vi "GetPublicEvents.vi"(8 "error in (no error)":errorcluster, 11 "SMO":refnum<class "SMO.lvclass">) -> (0 "error out":errorcluster, 2 "Public Events":T1, 3 "SMO out":refnum<class "SMO.lvclass">)   [LabVIEW 2013, in "SMO.lvclass"]
uses:
  SMO.lvclass
  Typedefs/Public Events.ctl
  SMO.lvclass/SMO.ctl
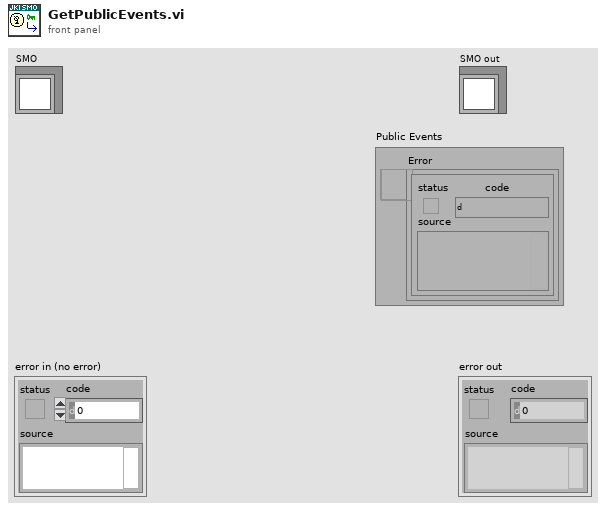
[diagram p1: front panel]
types:
  T1 = typedef "SMO.lvclass/Public Events.ctl" = cluster{"Error":refnum<user-event>}
  T2 = typedef "SMO.lvclass/PrivateData--Ref.ctl" = refnum<data-value>
  T3 = typedef "SMO.lvclass/PrivateData--Cluster.ctl" = cluster{"SMO Name":string, "Parent Call":T4, "Registered Processes":T5[], "Process Sync RendezVous":T6, "Process Error Notifier":refnum<notifier>, "Protected Events":T7, "Public Events":T1}
  T4 = typedef "SMO.lvclass/Parent Call--Enum.ctl" = enum16{"Allows parent to run", "Does not request parent to run"}
  T5 = typedef "SMO.lvclass/RegisteredProcessData--Cluster.ctl" = cluster{"Name":string, "Static VI Ref":refnum<vi>, "Running":bool}
  T6 = typedef "Rendezvous RefNum" = refnum<k1>
  T7 = typedef "SMO.lvclass/Protected Events.ctl" = cluster{"StopProcesses":refnum<user-event>, "AbortProcesses":refnum<user-event>}
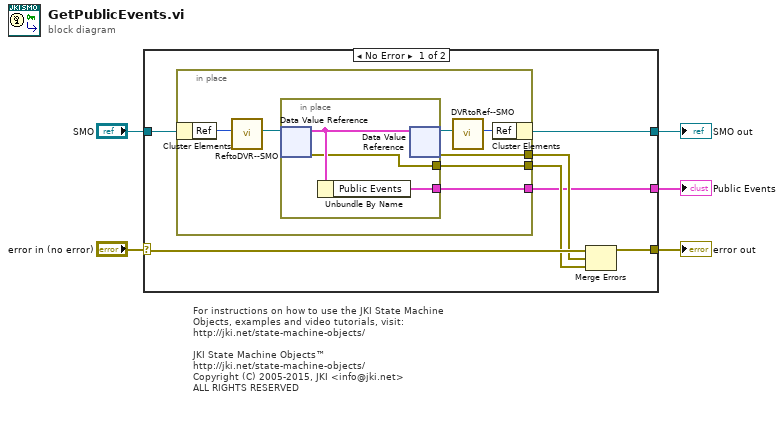
[diagram p0: block diagram]
diagram:
  # "For instructions on how to use the JKI State Machine Objects, examples and video tutorials, visit:\nhttp://jki.net/state-machine-objects/\n\nJKI State Machine Objects™\nhttp://jki.net/state-machine-objects/\nCopyright (C) 2005-2015, JKI <info@jki.net>\nALL RIGHTS RESERVED"
  n1 = case shown="No Error" "error in (no error)" {
    selector: "error in (no error)" -> [w10 w24]
    tunnel: [w9 w24] -> w4
    tunnel: [w11 w23] -> w2
    tunnel: "SMO" -> [w12 w23]
    tunnel: [w6 _] -> w1
    frame No Error {
      n2 = in-place {
        in-place-border: [w19] -> w6
        in-place-border: [w18] -> w8
        in-place-border: [w17] -> w7
        n3 = in-place-cluster #1(w12) -> ("Ref"=w16:u32)
        n4 = call "ReftoDVR--SMO.vi"("Ref"=w16) -> ("Ref"=w15:T2)  [unwired: 10 in]
        n5 = in-place {
          in-place-border: [w22] -> w19
          in-place-border: [w20] -> w17
          n6 = in-place-dvr #2(w15) -> (w21:T3, w20:errorcluster)
          n7 = Unbundle By Name(w21) -> ("Public Events"=w22:T1)
          n8 = in-place-dvr #2(w21) -> (w14:T2, w18:errorcluster)
        }
        n9 = call "DVRtoRef--SMO.vi"("Ref"=w14) -> ("Ref"=w13:u32)  [unwired: 10 in]
        n10 = in-place-cluster #1("Ref"=w13) -> (w11:refnum<class "SMO.lvclass">)
      }
      n11 = Merge Errors(w10, w8, w7) -> (w9:errorcluster)
    }
    frame Error {
    }
  }
  "error out" <- w4
  "SMO out" <- w2
  "Public Events" <- w1
